vi "TP 2.4.vi"() -> ()   [LabVIEW 2013]
panel:
  in  "Función":T1(ring)
  in  "stop":bool
  out "Waveform Graph":dbl[](graph)
  in  "Amplitud":dbl
  in  "Frecuencia":dbl
  in  "Cantida de Muestras":dbl
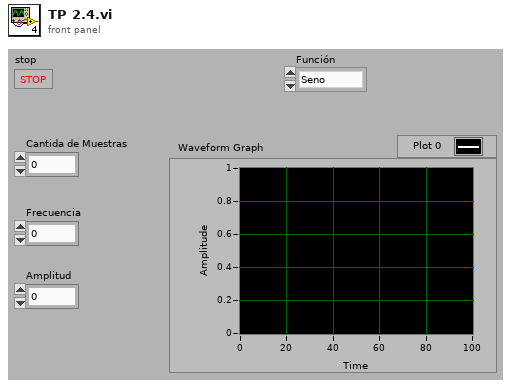
[diagram p1: front panel]
types:
  T1 = enum16{"Seno", "Rampa", "Triangular", "Cuadrada"}
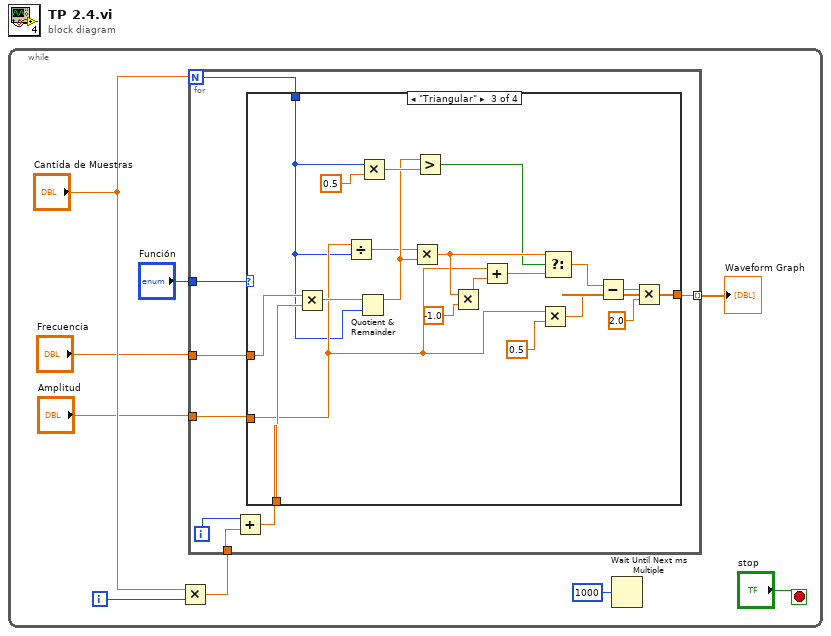
[diagram p0: block diagram]
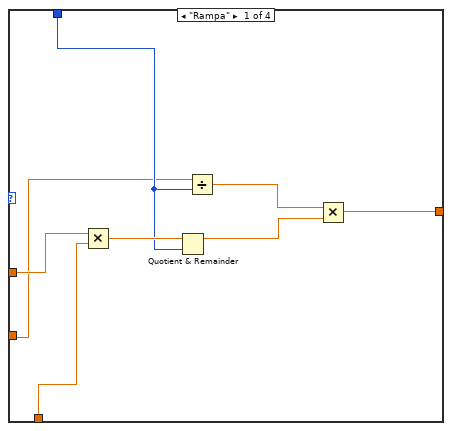
[diagram p2: hidden frame]
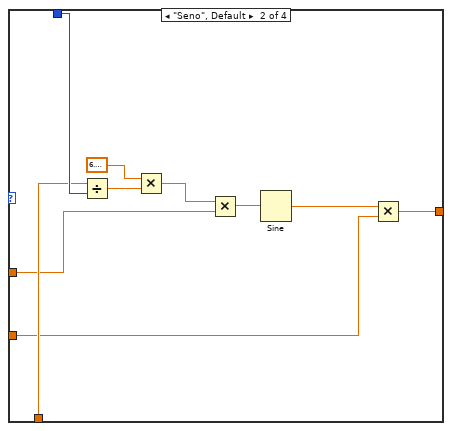
[diagram p3: hidden frame]
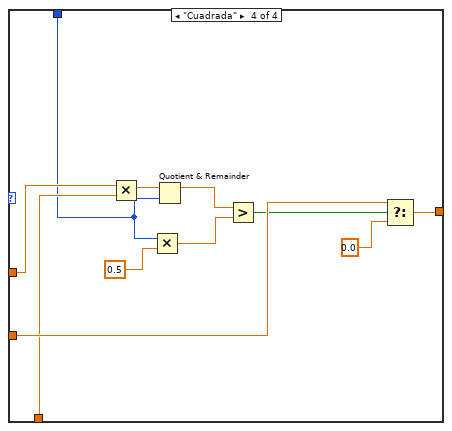
[diagram p4: hidden frame]
diagram:
  n1 = while {
    i -> [w6]
    stop <- "stop" stop-if-true
    n2 = Multiply(x="Cantida de Muestras", y=w6) -> (x*y=w5:dbl)
    n3 = for {
      N: "Cantida de Muestras" -> [w17]
      tunnel: "Frecuencia" -> [w16]
      tunnel: "Amplitud" -> [w15]
      tunnel: [w14] -> w9 mode=indexing
      tunnel: w5 -> [w13]
      tunnel: "Función" -> [w10]
      i -> [w12]
      n4 = Add(x=w12, y=w13) -> (x+y=w11:dbl)
      n5 = case shown="\"Triangular\"" w10 {
        tunnel: w17 -> [w22 w35 w36 w56]
        tunnel: w16 -> [w24 w27 w53 w65]
        tunnel: w15 -> [w21 w29 w44 w64]
        tunnel: [w19 w31 w40 w62] -> w14
        tunnel: w11 -> [w25 w30 w54 w58]
        frame "Rampa" {
          n6 = Multiply(x=w24, y=w25) -> (x*y=w23:dbl)
          n7 = Quotient & Remainder(x=w23, y=w22) -> (x-y*floor(x/y)=w18:dbl)  [unwired: 1 out]
          n8 = Divide(x=w21, y=w22) -> (x/y=w20:dbl)
          n9 = Multiply(x=w20, y=w18) -> (x*y=w19:dbl)
        }
        frame "Seno", Default {
          n10 = Divide(x=w30, y=w35) -> (x/y=w34:dbl)
          n11 = Multiply(x=6.283185307179586, y=w34) -> (x*y=w28:dbl)
          n12 = Multiply(x=w28, y=w27) -> (x*y=w33:dbl)
          n13 = Sine(x=w33) -> (sin(x)=w32:dbl)
          n14 = Multiply(x=w32, y=w29) -> (x*y=w31:dbl)
        }
        frame "Triangular" {
          n15 = Multiply(x=w53, y=w54) -> (x*y=w55:dbl)
          n16 = Divide(x=w44, y=w36) -> (x/y=w37:dbl)
          n17 = Quotient & Remainder(x=w55, y=w36) -> (x-y*floor(x/y)=w47:dbl)  [unwired: 1 out]
          n18 = Multiply(x=w36, y=0.5 ("x")) -> (x*y=w49:dbl)
          n19 = Multiply(x=w37, y=w47) -> (x*y=w52:dbl)
          n20 = Greater?(x=w47, y=w49) -> (0:w46:bool)
          n21 = Multiply(x=w52, y=-1.0) -> (x*y=w48:dbl)
          n22 = Add(x=w44, y=w48) -> (x+y=w39:dbl)
          n23 = Multiply(x=w44, y=0.5 ("x")) -> (x*y=w43:dbl)
          n24 = Select(t=w52, s=w46, f=w39) -> (s? t:f=w45:dbl)
          n25 = Subtract(x=w45, y=w43) -> (x-y=w42:dbl)
          n26 = Multiply(x=w42, y=2.0 ("x")) -> (x*y=w40:dbl)
        }
        frame "Cuadrada" {
          n27 = Multiply(x=w65, y=w58) -> (x*y=w66:dbl)
          n28 = Multiply(x=w56, y=0.5) -> (x*y=w57:dbl)
          n29 = Quotient & Remainder(x=w66, y=w56) -> (x-y*floor(x/y)=w60:dbl)  [unwired: 1 out]
          n30 = Greater?(x=w60, y=w57) -> (0:w63:bool)
          n31 = Select(t=w64, s=w63, f=0.0) -> (s? t:f=w62:dbl)
        }
      }
    }
    "Waveform Graph" <- w9
    n32 = Wait Until Next ms Multiple(millisecond multiple=u32 1000) -> ()  [unwired: 1 out]
  }
